vi "FW Quit.vi"(0 "Notifier Name In":string, 11 "Error In":errorcluster) -> (4 "Notifier Name Out":string, 15 "Error Out":errorcluster)   [LabVIEW 2020]
uses:
  FW Type Defs/FW Notifier Type.ctl
  FW Type Defs/FW Actions.ctl
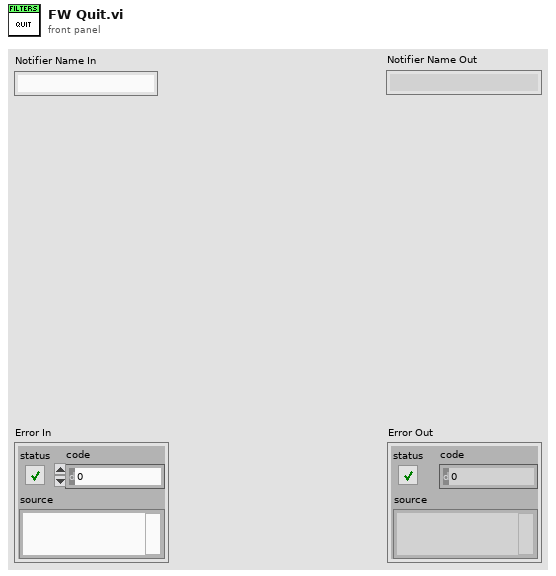
[diagram p1: front panel]
types:
  T1 = typedef "FW Notifier Type.ctl" = cluster{"Actions":T2, "Set Position":u8, "Actual Position":u8, "Speed":dbl, "Num Positions":u8, "Received":bool}
  T2 = typedef "FW Actions.ctl" = enum16{"Set Position", "Get Position", "Get Num Positions", "Set Speed", "Confirm Pos", "Quit"}
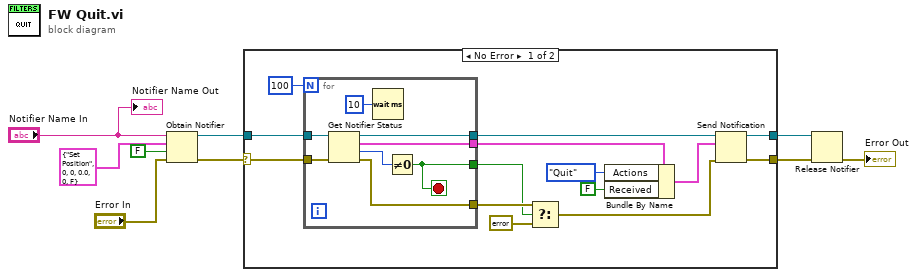
[diagram p0: block diagram]
diagram:
  n1 = Obtain Notifier(name (unnamed)="Notifier Name In", notification data type=T1 {"Actions"=enum."Set Position", "Set Position"=0, "Actual Position"=0, "Speed"=0.0, "Num Positions"=0, "Received"=FALSE} ("FW102C Note Type"), create if not found? (T)=FALSE, error in (no error)="Error In") -> (notifier out=w6:refnum<notifier>, error out=w7:errorcluster)  [unwired: 1 out]
  n2 = case shown="No Error" w7 {
    selector: w7 -> [w21 w33]
    tunnel: w6 -> [w23 w32]
    tunnel: [w11 w33] -> w3
    tunnel: [w12 w32] -> w4
    frame No Error {
      n3 = for {
        N: 100 -> [_]
        tunnel: w23 -> [w31]
        tunnel: [w29] -> w16
        tunnel: [w27] -> w20
        tunnel: w21 -> [w26]
        tunnel: [w25] -> w17
        tunnel: [w24] -> w13
        stop <- w29 stop-if-true
        n4 = Get Notifier Status(notifier=w31, error in (no error)=w26) -> (notifier out=w27:refnum<notifier>, current notification=w24:T1, # waiting=w30:i32, error out=w25:errorcluster)  [unwired: 1 out]
        n5 = Wait (ms)(milliseconds to wait=u32 10) -> ()  [unwired: 1 out]
        n6 = Not Equal To 0?(x=w30) -> (x != 0?=w29:bool)
      }
      n7 = Select(t=w17, s=w16, f=errorcluster {"status"=TRUE, "code"=0, "source"="Filter wheel busy. Timeout error."}) -> (s? t:f=w10:errorcluster)
      n8 = Bundle By Name(cluster=w13, "Actions"=FW_Actions."Quit", "Received"=FALSE) -> (w19:T1)
      n9 = Send Notification(notification=w19, notifier=w20, error in (no error)=w10) -> (notifier out=w12:refnum<notifier>, error out=w11:errorcluster)
    }
    frame Error {
    }
  }
  n10 = Release Notifier(notifier=w4, error in (no error)=w3) -> (error out=→"Error Out":errorcluster)  [unwired: 1 in, 2 out]
  "Notifier Name Out" <- "Notifier Name In"
